vi "Rinocloud_HTTP_update_metadata.vi"(5 "Extra metadata array":T1(array[cluster])=[{"Attribute"="", "Value"="", "Data type"=enum."<null>"}], 6 "parent ID":string, 7 "self ID":string, 8 "error in (no error)":errorcluster, 9 "Notes":string, 10 "Tags":string, 11 "Name":string) -> (0 "error out":errorcluster, 3 "Status":T2={"headers"="", "body"="", "ID"="", "Saved"=TRUE})   [LabVIEW 2011, in "Rinocloud Library.lvlib"]
uses:
  Rinocloud Library.lvlib
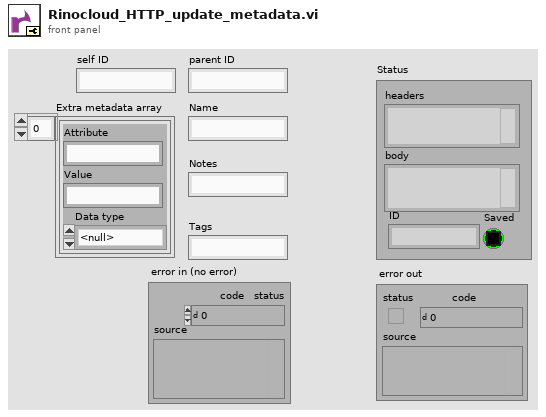
[diagram p1: front panel]
types:
  T1 = cluster{"Attribute":string, "Value":string, "Data type":enum16{"Numeric", "String", "1D array of strings", "1D array of doubles", "Data JSON string", "<null>"}}[]
  T2 = cluster{"headers":string, "body":string, "ID":string, "Saved":bool}
  T3 = cluster{"Name":string, "Notes":string, "Tags":string}
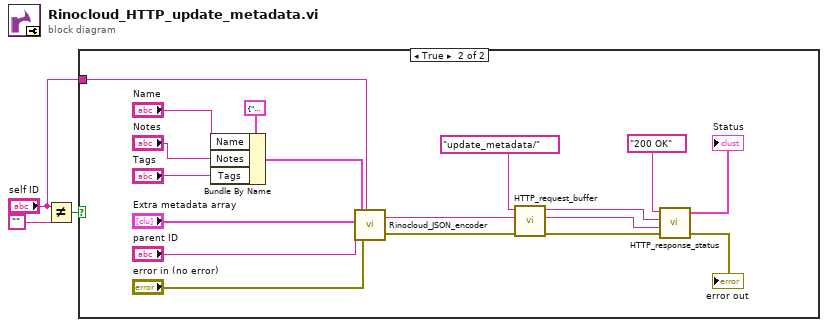
[diagram p0: block diagram]
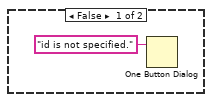
[diagram p2: hidden frame]
diagram:
  n1 = Not Equal?(x="self ID", y="") -> (x != y?=w2:bool)
  n2 = case shown="True" w2 {
    tunnel: "self ID" -> [_ w5]
    frame False {
      n3 = One Button Dialog(message="id is not specified.") -> ()  [unwired: 1 in, 1 out]
    }
    frame True {
      n4 = Bundle By Name(cluster=T3 {"Name"="", "Notes"="", "Tags"=""} ("Metadata"), "Name"="Name", "Notes"="Notes", "Tags"="Tags") -> (w14:T3)
      n5 = call "Rinocloud_JSON_encoder.vi"("Metadata"=w14, "Extra metadata array"="Extra metadata array", "parent ID"="parent ID", "error in (no error)"="error in (no error)", "self ID"=w5) -> ("JSON payload"=w17:string, "error out"=w20:errorcluster)
      n6 = call "HTTP_request_buffer.vi"("error in (no error)"=w20, "JSON payload"=w17, "Endpoint"="update_metadata/") -> ("error out"=w21:errorcluster, "body"=w19:string, "headers"=w18:string)  [unwired: 2 in]
      n7 = call "HTTP_response_status.vi"("error in (no error)"=w21, "body"=w19, "headers"=w18, "HTTP status"="200 OK") -> ("error out"=→"error out":errorcluster, "Status"=→"Status":T2)  [unwired: 1 in]
    }
  }
